vi "Sets the Number of Trigger Count.vi"(5 "Enable to Query":bool=TRUE, 7 "Enable to Sets":bool=TRUE, 8 "error in":errorcluster, 10 "Number of Trigger Count":u16=1 min=1 max=9999, 11 "VISA resource name":refnum<visa-resource-name>) -> (0 "error out":errorcluster, 2 "Return the Trigger Count":string, 3 "VISA resource name out":refnum<visa-resource-name>)   [LabVIEW 2011, in "DMM4.lvlib"]
uses:
  <instrlib>/DMM4/DMM4.lvlib
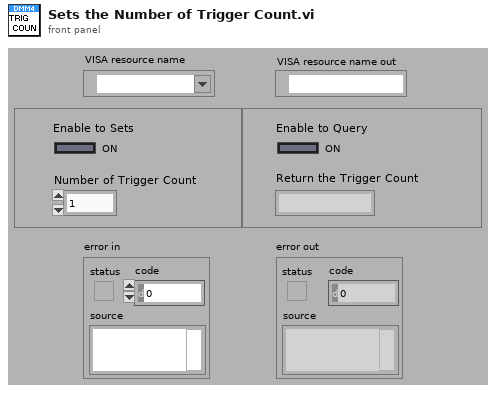
[diagram p1: front panel]
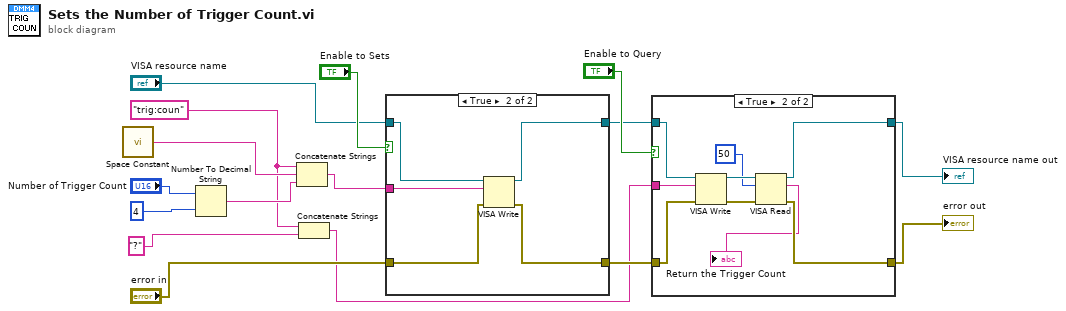
[diagram p0: block diagram]
diagram:
  w12 = "trig:coun"
  n1 = call <vilib>:"Space Constant.vi"() -> ("String"=w14:string)
  n2 = Number To Decimal String(number="Number of Trigger Count", width (-)=i16 4) -> (decimal integer string=w13:string)
  n3 = Concatenate Strings(w12, w14, w13) -> (w7:string)
  n4 = Concatenate Strings(w12, "?") -> (w1:string)
  n5 = case shown="True" "Enable to Sets" {
    tunnel: "VISA resource name" -> [w18 w23]
    tunnel: "error in" -> [w17 w22]
    tunnel: [w18 w21] -> w5
    tunnel: [w17 w20] -> w4
    tunnel: w7 -> [_ w19]
    frame False {
    }
    frame True {
      n6 = VISA Write(VISA resource name=w23, write buffer=w19, error in (no error)=w22) -> (VISA resource name out=w21:refnum<visa-resource-name>, error out=w20:errorcluster)  [unwired: 1 out]
    }
  }
  n7 = case shown="True" "Enable to Query" {
    tunnel: w5 -> [w25 w34]
    tunnel: w4 -> [w24 w33]
    tunnel: [w25 w30] -> w3
    tunnel: [w24 w29] -> w2
    tunnel: w1 -> [_ w27]
    frame False {
    }
    frame True {
      n8 = VISA Write(VISA resource name=w34, write buffer=w27, error in (no error)=w33) -> (VISA resource name out=w31:refnum<visa-resource-name>, error out=w32:errorcluster)  [unwired: 1 out]
      n9 = VISA Read(VISA resource name=w31, byte count=u32 50, error in (no error)=w32) -> (VISA resource name out=w30:refnum<visa-resource-name>, read buffer=→"Return the Trigger Count":string, error out=w29:errorcluster)  [unwired: 1 out]
    }
  }
  "VISA resource name out" <- w3
  "error out" <- w2
